vi "WriteDeviceTypeConfig.vi"(8 "error in (no error)":errorcluster, 11 "body":u8[](array[numeric])) -> (0 "error out":errorcluster, 3 "key values":T1[](array[typedef]))   [LabVIEW 2017, in "ServerComm.lvlib"]
uses:
  <vilib>/addons/InsightCM/Devices/Shared/Common/ServerComm/ServerComm.lvlib
  <vilib>/addons/InsightCM/MessageBus/Base/controls/SectionKeyValues.ctl
  <vilib>/addons/InsightCM/MessageBus/Base/controls/KeyValuePair.ctl
  <vilib>/addons/InsightCM/Utilities/GlobalConfiguration/GlobalConfiguration.lvlib
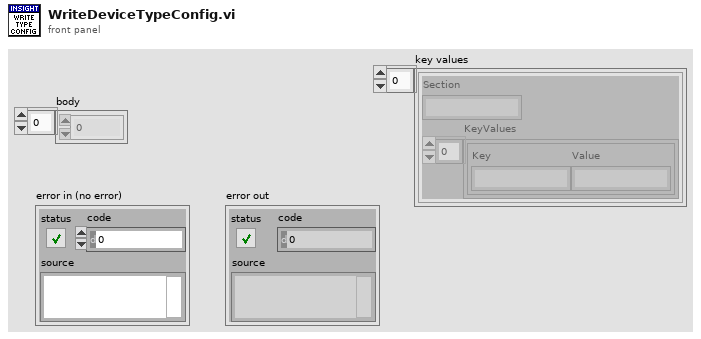
[diagram p1: front panel]
types:
  T1 = typedef "SectionKeyValues.ctl" = cluster{"Section":string, "KeyValues":T2[]}
  T2 = typedef "KeyValuePair.ctl" = cluster{"Key":string, "Value":string}
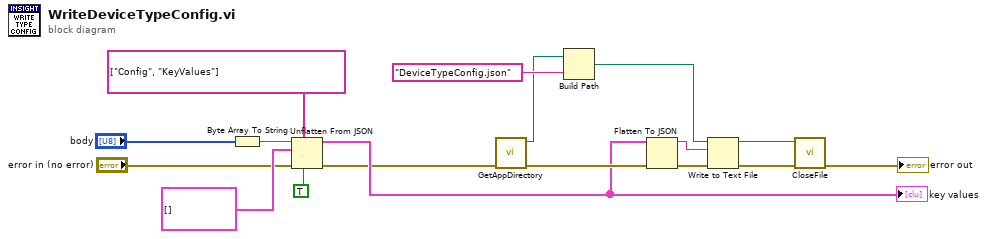
[diagram p0: block diagram]
diagram:
  n1 = Byte Array To String(unsigned byte array="body") -> (string=w7:string)
  n2 = Unflatten From JSON(path=string[] ["Config", "KeyValues"], JSON string=w7, type and defaults=T1[] [] ("KeyValues"), default null elements? (F)=TRUE, error in (no error)="error in (no error)") -> (value=w3:T1[], error out=w1:errorcluster)  [unwired: 2 in]
  "key values" <- w3
  n3 = call <vilib>:"GetAppDirectory.vi"("error in (no error)"=w1) -> ("error out"=w12:errorcluster, "application directory"=w16:path)  [unwired: 9 in]
  n4 = Build Path(base path=w16, name or relative path="DeviceTypeConfig.json") -> (appended path=w13:path)
  n5 = Flatten To JSON(anything=w3, error in (no error)=w12) -> (JSON string=w14:string, 11:w15:errorcluster)  [unwired: 1 in]
  n6 = Write to Text File(file (use dialog)=w13, text=w14, error in=w15) -> (refnum out=w11:refnum<file>, error out=w10:errorcluster)  [unwired: 1 in, 1 out]
  n7 = call <vilib>:"CloseFile.vi"("error in (no error)"=w10, "file reference"=w11) -> ("error out"=→"error out":errorcluster)  [unwired: 9 in]
